vi "GaussianFit.vi"(0 "Initial guess coefficients":dbl[](array[numeric])=[1.0, 1.0, 4.0, 1.0] format="%.2f", 1 "Input gaussian":dbl[](array[numeric])=[7.831458144390163e-10, 3.574868398677128e-08, 1.1114805454889874e-06, 2.3537918318837624e-05, 0.0003395147263754942, 0.003335596892793892, 0.02232096075549141, 0.1017364516552175, 0.31583820870842033, 0.6678472293163922, 0.9618646596277881, 0.9435723093822073, 0.6304647147873671, 0.28692656733953087, 0.08894163710163848, 0.01877862781601397, 0.0027005173331770306, 0.0002645175325415944, 1.764762780573516e-05, 8.01941313985562e-07] format="%.2f", 2 "Input abscissae":dbl[](array[numeric])=[-10.0, -8.947368421052632, -7.894736842105264, -6.842105263157896, -5.789473684210527, -4.736842105263159, -3.684210526315791, -2.631578947368423, -1.5789473684210547, -0.5263157894736863, 0.5263157894736821, 1.5789473684210504, 2.6315789473684186, 3.6842105263157867, 4.736842105263155, 5.789473684210523, 6.842105263157891, 7.894736842105259, 8.947368421052628, 9.999999999999996] format="%.2f") -> (3 "Amplitude":dbl=0.9999608042664722 format="%.2f", 4 "Central abscissa":dbl=1.000000015511602 format="%.2f", 5 "FWHM":dbl=4.000130102505921 format="%.2f", 6 "Best fit gaussian":dbl[](array[numeric])=[5.057069539451424e-10, 2.4984484875520733e-08, 8.340915380897895e-07, 1.881606793430916e-05, 0.0002868242529060693, 0.0029544368479824915, 0.020563895723314157, 0.09671813560159996, 0.3073847242009499, 0.6601285063495098, 0.9579581467914834, 0.9393694338021736, 0.6224409479599132, 0.2786966368368249, 0.08432127055775102, 0.017239092398355103, 0.0023815707867776517, 0.00022232301991877308, 1.4024171470768972e-05, 5.977806250361027e-07] format="%.2f")   [LabVIEW 2009]
uses:
  <vilib>/gmath/NI_Gmath.lvlib
panel:
  out "Zero level":dbl=4.000130102505921 format="%.2f"
  in  "model description":T1={"model"="a*exp(-(x-b)*(x-b)/(c*c))+d", "Parameters"=["a", "b", "c", "d"], "x"="x"}
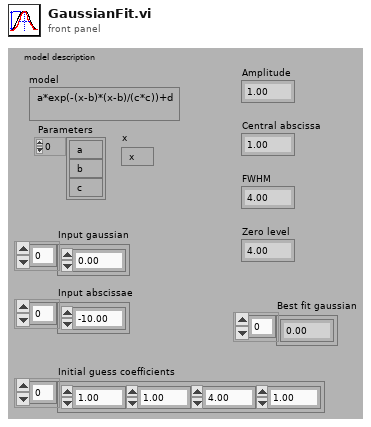
[diagram p1: front panel]
types:
  T1 = cluster{"model":string, "Parameters":string[], "x":string}
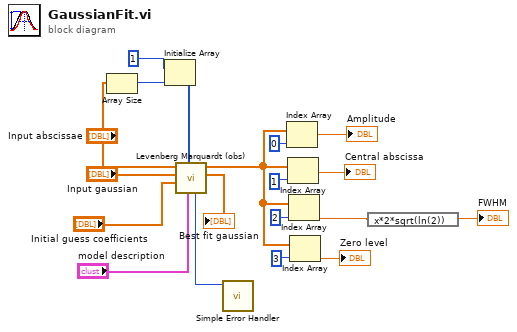
[diagram p0: block diagram]
diagram:
  n1 = Array Size(array="Input abscissae") -> (size(s)=w7:i32)
  n2 = Initialize Array(1, w7) -> (w5:i32[])
  n3 = call <vilib>:"Levenberg Marquardt (obs).vi"("model description"="model description", "Standard Deviation"=w5, "Initial Guess Coefficient"="Initial guess coefficients", "Y"="Input gaussian", "X"="Input abscissae") -> ("Best Fit"=→"Best fit gaussian":dbl[], "Best Fit Coefficients"=w3:dbl[], "error"=w9:i32)  [unwired: 1 in, 3 out]
  n4 = call <vilib>:"Simple Error Handler.vi"("error code (no error:0)"=w9) -> ()  [unwired: 4 in, 5 out]
  n5 = Index Array(array=w3, index=0) -> (element=→"Amplitude":dbl)
  n6 = Index Array(array=w3, index=1) -> (element=→"Central abscissa":dbl)
  n7 = Index Array(array=w3, index=2) -> (element=w11:dbl)
  n8 = Index Array(array=w3, index=3) -> (element=→"Zero level":dbl)
  n9 = expression code="x*2*sqrt(ln(2))"(w11) -> (→"FWHM":dbl)
